vi "Save.vi"(8 "error in":errorcluster, 11 "Datawarehouse in":refnum<class "Datawarehouse.lvclass">) -> (0 "error out":errorcluster, 3 "Datawarehouse out":refnum<class "Datawarehouse.lvclass">)   [LabVIEW 2021, in "ProligentXMLGenerator.lvlib" / "Datawarehouse.lvclass"]
doc: "Saves the ProligentCanonicalFile on disk."
uses:
  Datawarehouse.lvclass
  Datawarehouse.lvclass/Datawarehouse.ctl
  Base/DateTime/DateTime.lvclass
  ProligentXMLGenerator.lvlib
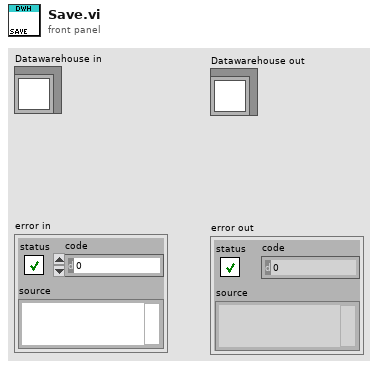
[diagram p1: front panel]
types:
  T1 = typedef "ProligentXMLGenerator.lvlib/Datawarehouse.lvclass/Data.ctl" = cluster{"DestinationFolder":path, "BaseFileName":string, "Document":refnum<k20>, "Defects":refnum<class "Defect.lvclass">[], "TopProcessRuns":refnum<class "ProcessRun.lvclass">[], "ProductUnits":refnum<class "ProductUnit.lvclass">[], "GenerationTime":refnum<class "DateTime.lvclass">, "DataSourceFingerprint":refnum<class "NonEmptyString_448.lvclass">, "IntegrationMetaData":refnum<class "NonEmptyString_2000.lvclass">, "TimeZoneInfoId":string}
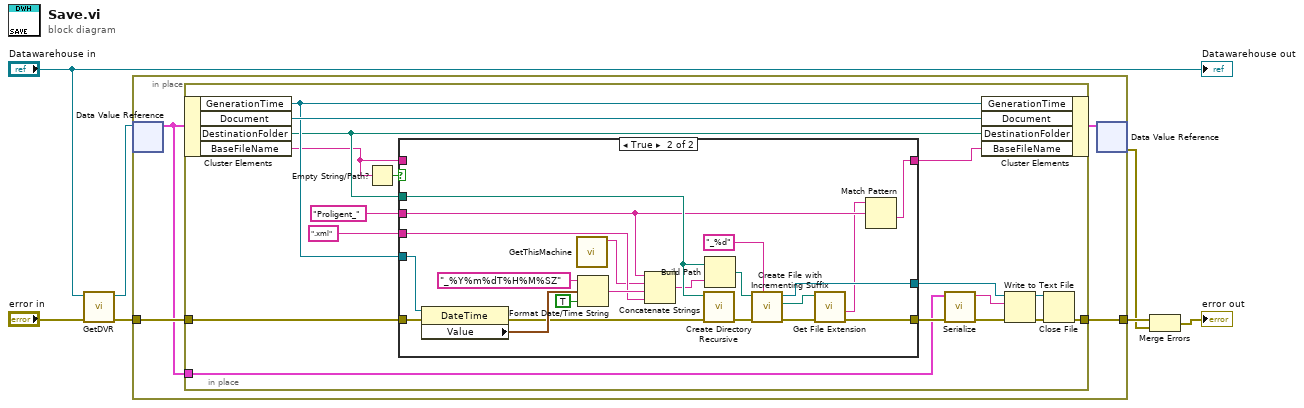
[diagram p0: block diagram]
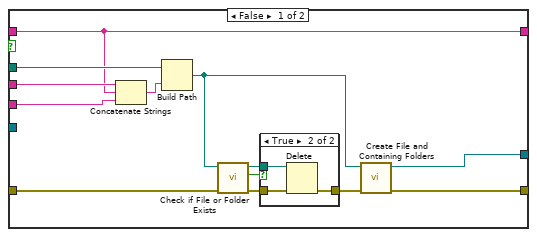
[diagram p2: hidden frame]
diagram:
  n1 = call "GetDVR.vi"("error in"="error in", "Datawarehouse"="Datawarehouse in") -> ("error out"=w4:errorcluster, "DVRReference"=w3:refnum<data-value>)  [unwired: 8 in]
  n2 = in-place "In Place Element Structure" {
    in-place-border: [w11] -> w5
    in-place-border: w4 -> [w10]
    n3 = in-place-dvr #1(w3) -> (w8:T1)  [unwired: 1 out]
    n4 = in-place "In Place Element Structure" {
      in-place-border: [w26] -> w11
      in-place-border: w10 -> [w13]
      in-place-border: w8 -> [w12]
      n5 = in-place-cluster #2(w8) -> ("GenerationTime"=w22:refnum<class "DateTime.lvclass">, "Document"=w23:refnum<k20>, "DestinationFolder"=w21:path, "BaseFileName"=w20:string)
      n6 = Empty String/Path?(string/path=w20) -> (empty?=w25:bool)
      n7 = case shown="True" w25 {
        tunnel: w22 -> [_ w64]
        tunnel: w13 -> [w35 w62]
        tunnel: [w38 w53] -> w24
        tunnel: [w36 w50] -> w16
        tunnel: w21 -> [w34 w57]
        tunnel: w20 -> [w30 _]
        tunnel: [w30 w47] -> w19
        tunnel: "Proligent_" -> [w32 w49]
        tunnel: ".xml" -> [w31 w56]
        frame False {
          n8 = Concatenate Strings(w32, w30, w31) -> (w29:string)
          n9 = Build Path(base path=w34, name or relative path=w29) -> (appended path=w33:path)
          n10 = call <vilib>:"Check if File or Folder Exists.vi"("error in (no error)"=w35, "path"=w33) -> ("error out"=w39:errorcluster, "file or folder exists?"=w41:bool, "dup path"=w40:path)  [unwired: 7 in]
          n11 = case shown="True" w41 {
            tunnel: w39 -> [w42 w45]
            tunnel: [w42 w44] -> w37
            tunnel: w40 -> [_ w43]
            frame False {
            }
            frame True {
              n12 = Delete(path (use dialog)=w43, error in=w45) -> (error out=w44:errorcluster)  [unwired: 3 in, 2 out]
            }
          }
          n13 = call <vilib>:"Create File and Containing Folders.vi"("error in (no error)"=w37, "file path"=w33) -> ("error out"=w36:errorcluster, "refnum out"=w38:refnum<file>)  [unwired: 8 in]
        }
        frame True {
          n14 = property on="Property Node" class="DateTime"(reference=w64, error in=w62) -> (error out=w60:errorcluster, "Value"=w63:timestamp)  [unwired: 1 out]
          n15 = call "GetThisMachine.vi"() -> ("ThisMachine"=w46:string)  [unwired: 11 in]
          n16 = Format Date/Time String(time format string (%c)="_%Y%m%dT%H%M%SZ", seconds (now)=w63, UTC format=TRUE) -> (date/time string=w65:string)
          n17 = Concatenate Strings(w49, w46, w65, w56) -> (w55:string)
          n18 = call <vilib>:"Create Directory Recursive.vi"("error in (no error)"=w60, "directory"=w57) -> ("error out"=w59:errorcluster)  [unwired: 3 in, 2 out]
          n19 = Build Path(base path=w57, name or relative path=w55) -> (appended path=w61:path)
          n20 = call <vilib>:"Create File with Incrementing Suffix.vi"("format string (\" (%d)\")"="_%d" ("format string (\" (%d)\")"), "error in (no error)"=w59, "file path"=w61) -> ("error out"=w51:errorcluster, "actual path"=w52:path, "refnum out"=w53:refnum<file>)  [unwired: 6 in]
          n21 = call <vilib>:"Get File Extension.vi"("error in (no error)"=w51, "file"=w52) -> ("error out"=w50:errorcluster, "filename without extension"=w48:string)  [unwired: 5 in, 3 out]
          n22 = Match Pattern(string=w48, regular expression=w49) -> (after substring=w47:string)  [unwired: 1 in, 3 out]
        }
      }
      n23 = call "Serialize.vi"("error in"=w16, "Data"=w12) -> ("error out"=w14:errorcluster, "XMLString"=w15:string)  [unwired: 8 in]
      n24 = in-place-cluster #2("GenerationTime"=w22, "Document"=w23, "DestinationFolder"=w21, "BaseFileName"=w19) -> (w9:T1)
      n25 = Write to Text File(file (use dialog)=w24, text=w15, error in=w14) -> (refnum out=w27:refnum<file>, error out=w28:errorcluster)  [unwired: 1 in, 1 out]
      n26 = Close File(refnum=w27, error in=w28) -> (error out=w26:errorcluster)  [unwired: 1 out]
    }
    n27 = in-place-dvr #1(w9) -> (w2:errorcluster)  [unwired: 1 out]
  }
  n28 = Merge Errors(w5, w2) -> (→"error out":errorcluster)
  "Datawarehouse out" <- "Datawarehouse in"
